vi "Test TelegramTime to TimeStamp.vi"(11 "date":i64) -> (3 "time stamp":timestamp)   [LabVIEW 2015]
doc: "Created IvanLis by LabVIEW Portal\nProfile: http://labviewportal.org/memberlist.php?mode=viewprofile&u=987\neMail: IvanLisanov@gMail.com\nTelegram: https://t.me/IvanLis"
uses:
  Telegram Library/Telegram Library.lvlib
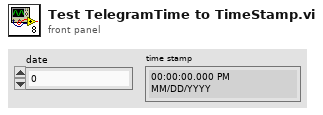
[diagram p1: front panel]
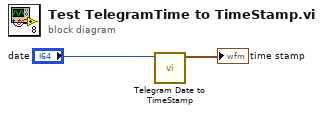
[diagram p0: block diagram]
diagram:
  n1 = call "Telegram Date to TimeStamp.vi"("date"="date") -> ("time stamp"=→"time stamp":timestamp)  [unwired: 10 in]
